vi "Set Frame Rate Enable.vi"(8 "error in (no error)":errorcluster, 10 "Enable":bool, 11 "Camera in":refnum<class "Camera.lvclass">) -> (0 "error out":errorcluster, 3 "Camera":refnum<class "Camera.lvclass">)   [LabVIEW 2020, in "Camera.lvclass"]
uses:
  Camera.lvclass
  Camera.lvclass/Camera.ctl
  Check Not Disconnected.vi
  <vilib>/Utility/error.llb/Error Cluster From Error Code.vi
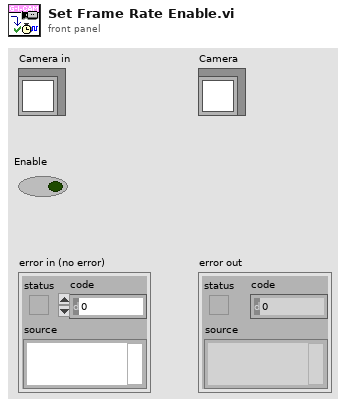
[diagram p1: front panel]
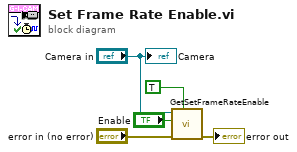
[diagram p0: block diagram]
diagram:
  n1 = call "GetSetFrameRateEnable.vi"("Set?"=TRUE, "error in (no error)"="error in (no error)", "Value in"="Enable", "Camera in"="Camera in") -> ("error out"=→"error out":errorcluster)  [unwired: 6 in, 1 out]
  "Camera" <- "Camera in"
